vi "Detector Send Data to Data Q.vi"(8 "error in (no error)":errorcluster, 10 "element":T1, 11 "Data Q":refnum<queue>) -> (0 "error out":errorcluster)   [LabVIEW 2021]
uses:
  Subsystems/SS cluster Data Queue type.ctl
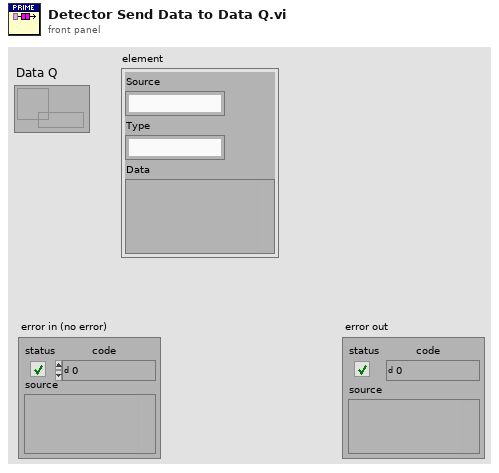
[diagram p1: front panel]
types:
  T1 = typedef "SS cluster Data Queue type.ctl" = cluster{"Source":string, "Type":string, "Data":variant}
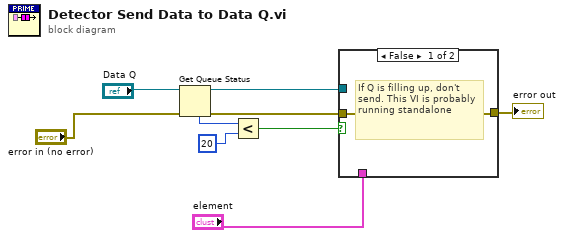
[diagram p0: block diagram]
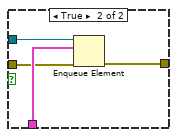
[diagram p2: hidden frame]
diagram:
  n1 = Get Queue Status(queue="Data Q", error in (no error)="error in (no error)") -> (queue out=w5:refnum<queue>, error out=w2:errorcluster, # elements in queue=w9:i32)  [unwired: 1 in, 5 out]
  n2 = Less?(x=w9, y=20) -> (x < y?=w4:bool)
  n3 = case shown="False" w4 {
    tunnel: "element" -> [_ w14]
    tunnel: w5 -> [_ w13]
    tunnel: w2 -> [w10 w12]
    tunnel: [w10 w11] -> w1
    frame False {
      # "If Q is filling up, don't send. This VI is probably running standalone"
    }
    frame True {
      n4 = Enqueue Element(queue=w13, element=w14, error in (no error)=w12) -> (error out=w11:errorcluster)  [unwired: 1 in, 2 out]
    }
  }
  "error out" <- w1
